vi "Write Pigeon speed [km_h].vi"(8 "error in (no error)":errorcluster, 10 "Pigeon speed [km/h]":dbl=70.0, 11 "Pigeon in":refnum<class "Pigeon.lvclass">) -> (0 "error out":errorcluster, 3 "Pigeon out":refnum<class "Pigeon.lvclass">)   [LabVIEW 2019, in "Pigeon.lvclass"]
uses:
  Pigeon.lvclass
  Pigeon.lvclass/Pigeon.ctl
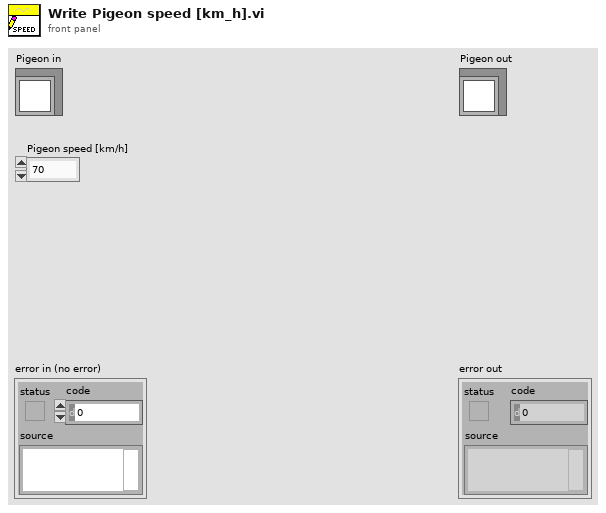
[diagram p1: front panel]
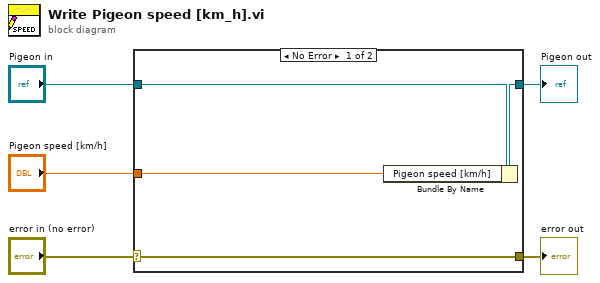
[diagram p0: block diagram]
diagram:
  n1 = case shown="No Error" "error in (no error)" {
    selector: "error in (no error)" -> [w9 w10]
    tunnel: [w9 w10] -> w4
    tunnel: [w7 w11] -> w2
    tunnel: "Pigeon in" -> [w8 w11]
    tunnel: "Pigeon speed [km/h]" -> [w6 _]
    frame No Error {
      n2 = Bundle By Name(cluster=w8, "Pigeon speed [km/h]"=w6) -> (w7:refnum<class "Pigeon.lvclass">)
    }
    frame Error {
    }
  }
  "error out" <- w4
  "Pigeon out" <- w2
